vi "模拟量输出测试.vi"() -> ()   [LabVIEW 2010]
panel:
  in  "停止":bool
  in  "数组":dbl[][](array[numeric])
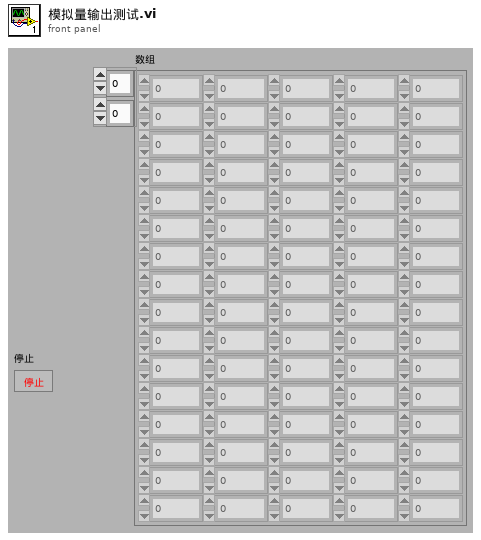
[diagram p1: front panel]
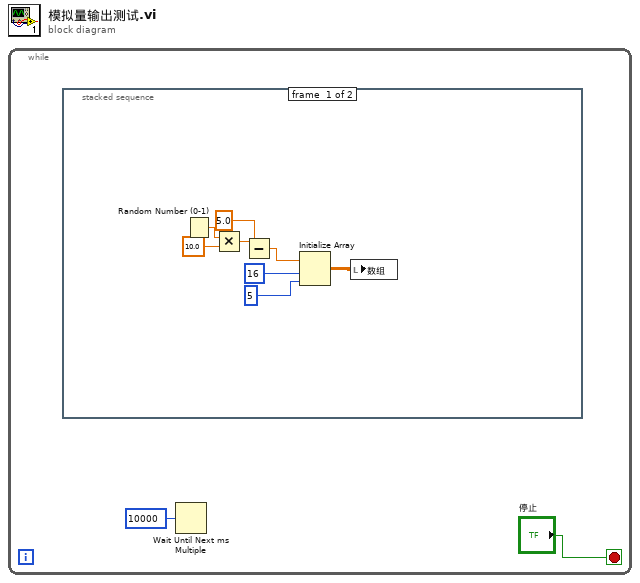
[diagram p0: block diagram]
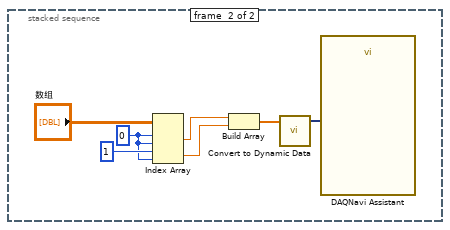
[diagram p2: hidden frame]
diagram:
  n1 = while {
    stop <- "停止" stop-if-true
    n2 = stacked-sequence {
      frame #0 {
        n3 = Random Number (0-1)() -> (number: 0 to 1=w7:dbl)
        n4 = Multiply(x=w7, y=10.0) -> (x*y=w5:dbl)
        n5 = Subtract(x=w5, y=5.0) -> (x-y=w3:dbl)
        n6 = Initialize Array(w3, 16 ("维数大小"), 5 ("维数大小")) -> (w10:dbl[][])
        n7 = local write "数组"(w10) -> ()
      }
      frame #1 {
        w11 = 0 ("索引 (行)")
        n8 = Index Array(array="数组", index (row) #1=w11, index (col) #1=w11, index (row) #2=1 ("禁用的索引 (列)"), index (col) #2=w11) -> (element #1=w14:dbl, element #2=w13:dbl)
        n9 = Build Array(w14, w13) -> (w15:dbl[])
        n10 = call "Convert to Dynamic Data"("Array"=w15) -> ("Dynamic Data Type"=w16:dynamicdata)  [unwired: 3 out]
        n11 = call "DAQNavi Assistant"("data in(DDT)"=w16) -> ()  [unwired: 2 in, 17 out]
      }
    }
    n12 = Wait Until Next ms Multiple(millisecond multiple=u32 10000 ("毫秒倍数")) -> ()  [unwired: 1 out]
  }
